vi "execute.vi"(8 "error in (no error)":errorcluster, 9 "image assembler in":refnum<class "GenericComponent.lvclass">, 10 "imaging mode in":refnum<class "GenericComponent.lvclass">, 11 "adapter in":refnum<class "AdapterTS090827ImagingModeToImageAssembler.lvclass">) -> (0 "error out":errorcluster, 1 "image assembler out":refnum<class "GenericComponent.lvclass">, 2 "imaging mode out":refnum<class "GenericComponent.lvclass">, 3 "adapter out":refnum<class "AdapterTS090827ImagingModeToImageAssembler.lvclass">)   [LabVIEW 2010, in "AdapterTS090827ImagingModeToImageAssembler.lvclass"]
uses:
  AdapterTS090827ImagingModeToImageAssembler.lvclass
  common/classes/GenericComponent/GenericComponent/GenericComponent.lvclass
  ImageAssembler/ImageAssemblerDL090211Frame/ImageAssemblerDL090211Frame/ImageAssemblerDL090211Frame.lvclass
  ImagingMode/ImagingModeTS090821Circular2D/ImagingModeTS090821Circular2D/ImagingModeTS090821Circular2D.lvclass
panel:
  # "imaging mode: ImagingModeTS090821Circular2D\nimage assembler: ImageAssemblerDL090211Frame"
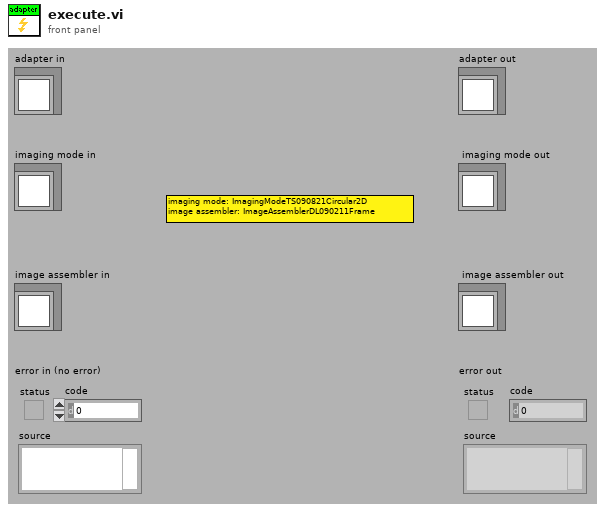
[diagram p1: front panel]
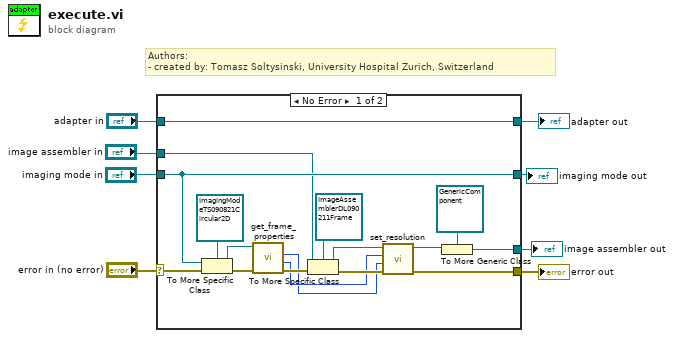
[diagram p0: block diagram]
diagram:
  # "Authors: \n- created by: Tomasz Soltysinski, University Hospital Zurich, Switzerland"
  n1 = case shown="No Error" "error in (no error)" {
    selector: "error in (no error)" -> [w25 w29]
    tunnel: [w23 w27] -> w2
    tunnel: "imaging mode in" -> [w23 w27]
    tunnel: [w24 w28] -> w6
    tunnel: "adapter in" -> [w24 w28]
    tunnel: [w21 w26] -> w1
    tunnel: "image assembler in" -> [w19 w26]
    tunnel: [w10 w29] -> w5
    frame No Error {
      n2 = To More Specific Class(target class=refnum<class "ImagingModeTS090821Circular2D.lvclass"> refnum ("ImagingModeTS090821Circular2D.lvclass"), reference=w23, error in=w25) -> (specific class reference=w17:refnum<class "ImagingModeTS090821Circular2D.lvclass">, error out=w18:errorcluster)
      n3 = call-dynamic "get_frame_properties.vi"("error in (no error)"=w18, "ScanModeTS090821Circular2D in"=w17) -> ("error out"=w16:errorcluster, "pixels per line"=w12:i32, "lines per frame"=w11:i32)  [unwired: 5 in, 2 out]
      n4 = To More Specific Class(target class=refnum<class "ImageAssemblerDL090211Frame.lvclass"> refnum ("ImageAssemblerDL090211Frame.lvclass"), reference=w19, error in=w16) -> (specific class reference=w13:refnum<class "ImageAssemblerDL090211Frame.lvclass">, error out=w14:errorcluster)
      n5 = call "set_resolution.vi"("error in (no error)"=w14, "y resolution"=w11, "x resolution"=w12, "DL090211FrameImageAssembler.lvclass in"=w13) -> ("error out"=w10:errorcluster, "DL090211FrameImageAssembler.lvclass out"=w9:refnum<class "ImageAssemblerDL090211Frame.lvclass">)  [unwired: 6 in]
      n6 = To More Generic Class(target class=refnum<class "GenericComponent.lvclass"> refnum ("GenericComponent.lvclass"), reference=w9) -> (generic class reference=w21:refnum<class "GenericComponent.lvclass">)
    }
    frame Error {
    }
  }
  "error out" <- w5
  "adapter out" <- w6
  "imaging mode out" <- w2
  "image assembler out" <- w1
